vi "MGCC_main_PhaseTwo.vi"   [LabVIEW 2016]
panel:
  # "Copyright <2020> <The University of Tennessee at Knoxville and the University of Tennessee Research Foundation>\n\nRedistribution and use in source and binary forms, with or without modification, are permitted provided that the following conditions are met:\n\n1. Redistributions of source code must retain the above copyright notice, this list of conditions and the following disclaimer.\n\n2. Redistributions in binary form must reproduce the above copyright notice, this list of conditions and the following disclaimer in the documentation and/or other materials provided with the distribution.\n\n3. Neither the name of the copyright holder nor the names of its contributors may be used to endorse or promote products derived from this software without specific prior written permission.\n\nTHIS SOFTWARE IS PROVIDED BY THE COPYRIGHT HOLDERS AND CONTRIBUTORS \"AS IS\" AND ANY EXPRESS OR IMPLIED WARRANTIES, INCLUDING, BUT NOT LIMITED TO, THE IMPLIED WARRANTIES OF MERCHANTABILITY AND FITNESS FOR A PARTICULAR PURPOSE ARE DISCLAIMED. IN NO EVENT SHALL THE COPYRIGHT HOLDER OR CONTRIBUTORS BE LIABLE FOR ANY DIRECT, INDIRECT, INCIDENTAL, SPECIAL, EXEMPLARY, OR CONSEQUENTIAL DAMAGES (INCLUDING, BUT NOT LIMITED TO, PROCUREMENT OF SUBSTITUTE GOODS OR SERVICES; LOSS OF USE, DATA, OR PROFITS; OR BUSINESS INTERRUPTION) HOWEVER CAUSED AND ON ANY THEORY OF LIABILITY, WHETHER IN CONTRACT, STRICT LIABILITY, OR TORT (INCLUDING NEGLIGENCE OR OTHERWISE) ARISING IN ANY WAY OUT OF THE USE OF THIS SOFTWARE, EVEN IF ADVISED OF THE POSSIBILITY OF SUCH DAMAGE."
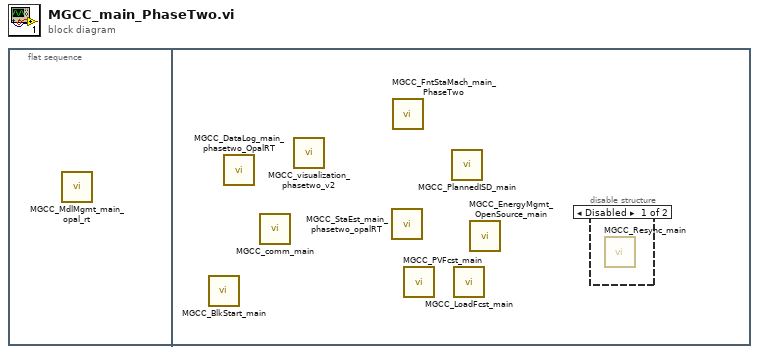
[diagram p0: block diagram]
diagram:
  n1 = flat-sequence {
    frame #0 {
      n2 = call "MGCC_MdlMgmt_main_opal_rt.vi"() -> ()  [unwired: 12 in]
    }
    frame #1 {
      n3 = call "MGCC_BlkStart_main.vi"() -> ()  [unwired: 12 in]
      n4 = call "MGCC_DataLog_main_phasetwo_OpalRT.vi"() -> ()  [unwired: 12 in]
      n5 = call "MGCC_comm_main.vi"() -> ()  [unwired: 12 in]
      n6 = call "MGCC_visualization_phasetwo_v2.vi"() -> ()  [unwired: 12 in]
      n7 = call "MGCC_StaEst_main_phasetwo_opalRT.vi"() -> ()  [unwired: 12 in]
      n8 = call "MGCC_FntStaMach_main_PhaseTwo.vi"() -> ()  [unwired: 12 in]
      n9 = call "MGCC_PVFcst_main.vi"() -> ()  [unwired: 12 in]
      n10 = call "MGCC_PlannedISD_main.vi"() -> ()  [unwired: 12 in]
      n11 = call "MGCC_LoadFcst_main.vi"() -> ()  [unwired: 12 in]
      n12 = call "MGCC_EnergyMgmt_OpenSource_main.vi"() -> ()  [unwired: 12 in]
      n13 = disable-structure shown="Disabled" {
        frame Disabled {
          n14 = call "MGCC_Resync_main.vi"() -> ()  [unwired: 12 in]
        }
        frame Enabled {
        }
      }
    }
  }
